vi "Disconnect.vi"(8 "error in (no error)":errorcluster, 11 "RSeries_CAM in":refnum<class "RSeries_CAM.lvclass">) -> (0 "error out":errorcluster, 3 "RSeries_CAM out":refnum<class "RSeries_CAM.lvclass">)   [LabVIEW 2024, in "RSeries_CAM.lvlib" / "RSeries_CAM.lvclass"]
uses:
  RSeries_CAM.lvclass
  RSeries_CAM.lvclass/RSeries_CAM.ctl
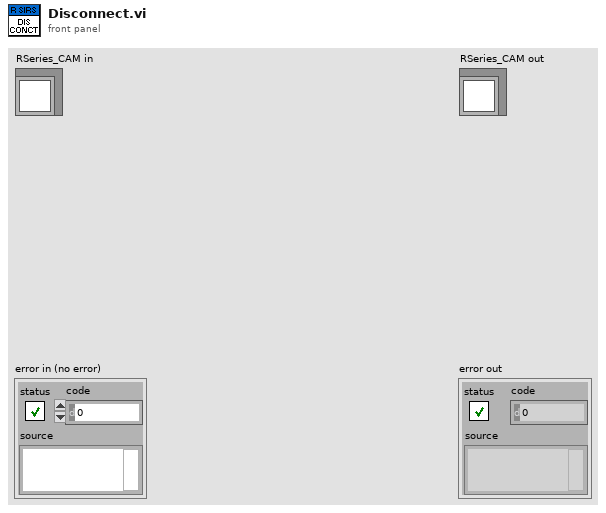
[diagram p1: front panel]
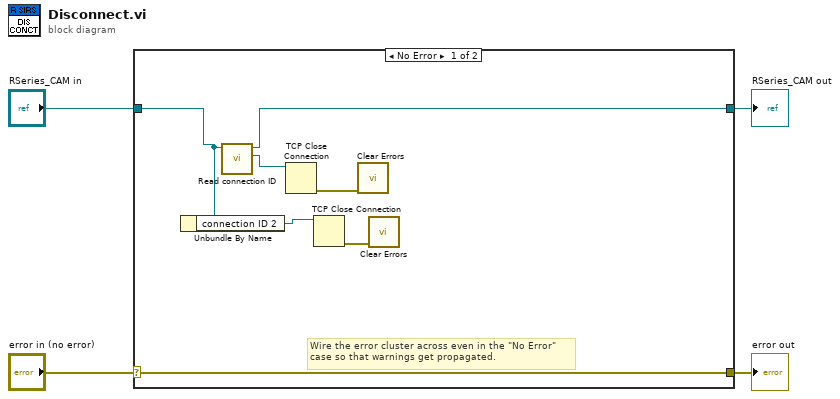
[diagram p0: block diagram]
diagram:
  n1 = case shown="No Error" "error in (no error)" {
    selector: "error in (no error)" -> [w11 w13]
    tunnel: [w11 w13] -> w3
    tunnel: [w8 w12] -> w1
    tunnel: "RSeries_CAM in" -> [w7 w12]
    frame No Error {
      # "Wire the error cluster across even in the \"No Error\"\ncase so that warnings get propagated."
      n2 = Unbundle By Name(w7) -> ("connection ID 2"=w6:refnum<k5>)
      n3 = call "Read connection ID.vi"("RSeries_CAM in"=w7) -> ("connection ID"=w10:refnum<k5>, "RSeries_CAM out"=w8:refnum<class "RSeries_CAM.lvclass">)  [unwired: 8 in, 1 out]
      n4 = TCP Close Connection(connection ID=w10) -> (error out=w9:errorcluster)  [unwired: 2 in, 1 out]
      n5 = TCP Close Connection(connection ID=w6) -> (error out=w5:errorcluster)  [unwired: 2 in, 1 out]
      n6 = call <vilib>:"Clear Errors.vi"("error in (no error)"=w9) -> ()  [unwired: 5 in, 2 out]
      n7 = call <vilib>:"Clear Errors.vi"("error in (no error)"=w5) -> ()  [unwired: 5 in, 2 out]
    }
    frame Error {
    }
  }
  "error out" <- w3
  "RSeries_CAM out" <- w1
